vi "From Hex String.vi"(8 "error in (no error)":errorcluster, 11 "String":string) -> (0 "error out":errorcluster, 3 "Packet out":refnum<class "Packet.lvclass">)   [LabVIEW 2020, in "Packet.lvclass"]
uses:
  Packet.lvclass
  Packet.lvclass/Packet.ctl
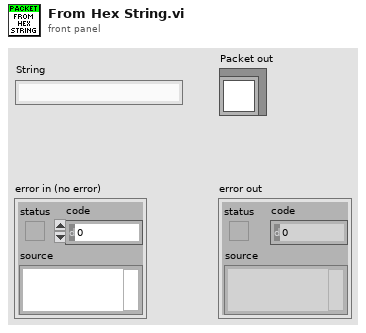
[diagram p1: front panel]
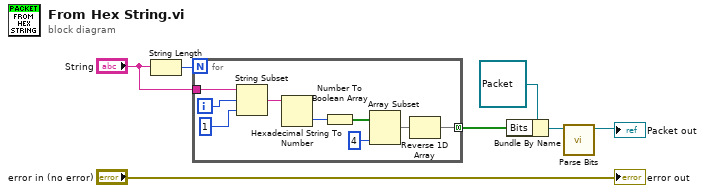
[diagram p0: block diagram]
diagram:
  n1 = String Length(string="String") -> (length=w5:i32)
  n2 = for {
    N: w5 -> [_]
    tunnel: "String" -> [w16]
    tunnel: [w8] -> w1 mode=concatenating
    i -> [w14]
    n3 = String Subset(string=w16, offset (0)=w14, length (rest)=1 ("length (rest)")) -> (substring=w13:string)
    n4 = Hexadecimal String To Number(string=w13) -> (number=w12:u32)  [unwired: 2 in, 1 out]
    n5 = Number To Boolean Array(number=w12) -> (Boolean array=w11:bool[])
    n6 = Array Subset(array=w11, length=4) -> (w9:bool[])  [unwired: 1 in]
    n7 = Reverse 1D Array(array=w9) -> (reversed array=w8:bool[])
  }
  n8 = Bundle By Name(cluster=refnum<class "Packet.lvclass"> refnum ("Packet.lvclass"), "Bits"=w1) -> (w2:refnum<class "Packet.lvclass">)
  n9 = call-dynamic "Parse Bits.vi"("Packet in"=w2) -> ("Packet out"=→"Packet out":refnum<class "Packet.lvclass">)  [unwired: 9 in, 1 out]
  "error out" <- "error in (no error)"
